vi "Process New Connection.vi"(8 "error in (no error)":errorcluster, 10 "New Connection Reference":refnum<data-value>, 11 "INewConnectionCallback in":refnum<class "INewConnectionCallback.lvclass">) -> (0 "error out":errorcluster)   [LabVIEW 2020, in "ConnectionFactorySession.lvlib" / "INewConnectionCallback.lvclass"]
uses:
  <vilib>/gpm_packages/@cs/Network-interface/Source/Connection Factory Session/INewConnectionCallback/INewConnectionCallback.lvclass
  <vilib>/gpm_packages/@cs/Network-interface/Source/Connection Reference/Connection Reference/Connection Reference.lvclass
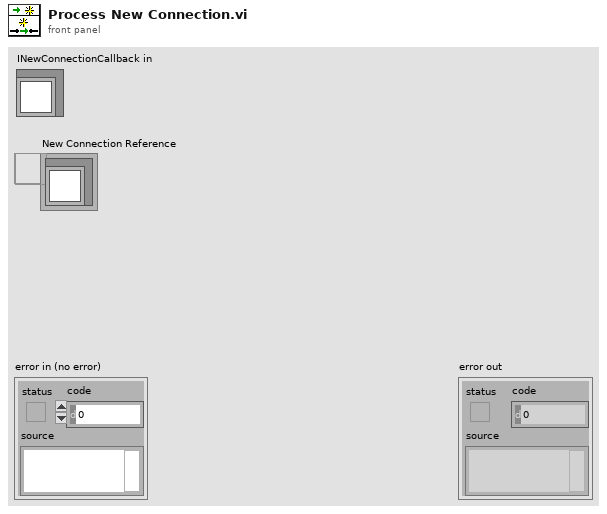
[diagram p1: front panel]
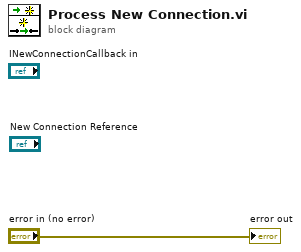
[diagram p0: block diagram]
diagram:
  "error out" <- "error in (no error)"
